vi "Translator.File.Order.vi"(8 "error in":errorcluster, 11 "Translation folder":path=path "D:/PL_0125_Sapphire_Automation_branches/SOFTWARE_v1.1-Translation/settings/Translation-Chinese.ini") -> (0 "error out":errorcluster)   [LabVIEW 2010]
uses:
  tma.lib/nlconfig.llb/nlRead Section (str).vi
  tma.lib/nlconfig.llb/nlWrite Section (str).vi
panel:
  out "section names":string[](array[string])
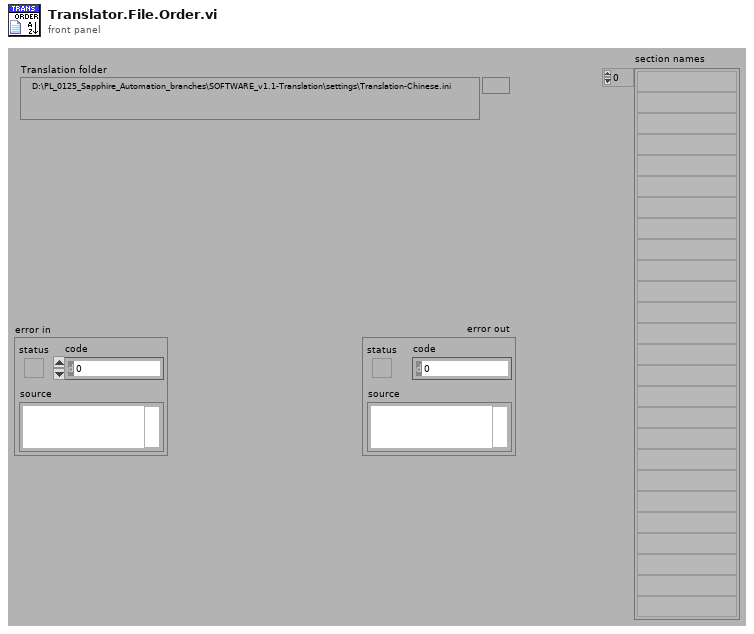
[diagram p1: front panel]
types:
  T1 = typedef "nlConfig Data RefNum.ctl" = refnum<k4>
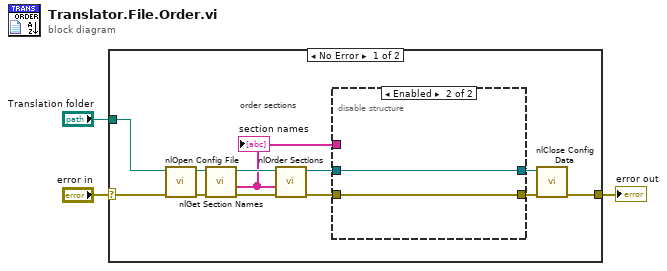
[diagram p0: block diagram]
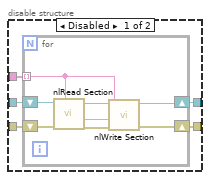
[diagram p2: hidden frame]
diagram:
  n1 = case shown="No Error" "error in" {
    selector: "error in" -> [w10 w31]
    tunnel: "Translation folder" -> [w11 _]
    tunnel: [w9 w31] -> w2
    frame No Error {
      # "order sections"
      n2 = call "nlOpen Config File.vi"("error in (no error)"=w10, "configuration file path"=w11) -> ("error out"=w12:errorcluster, "refnum"=w13:T1)  [unwired: 8 in]
      n3 = call "nlGet Section Names.vi"("error in (no error)"=w12, "refnum"=w13) -> ("error out"=w14:errorcluster, "section names"=w5:string[], "refnum out"=w15:T1)  [unwired: 7 in]
      "section names" <- w5
      n4 = call "nlOrder Sections.vi"("error in (no error)"=w14, "section names"=w5, "refnum"=w15) -> ("error out"=w8:errorcluster, "refnum out"=w7:T1)  [unwired: 7 in]
      n5 = disable-structure shown="Enabled" {
        disable-tunnel: w8 -> [w20 w29]
        disable-tunnel: w7 -> [w19 w30]
        disable-tunnel: [w18 w30] -> w6
        disable-tunnel: w5 -> [w17 _]
        disable-tunnel: [w16 w29] -> w4
        frame Disabled {
          n6 = for {
            tunnel: w17 -> [w23] mode=indexing
            shift-right: [w21] -> w18
            shift-left: w19 -> [w27]
            shift-right: [w22] -> w16
            shift-left: w20 -> [w28]
            n7 = call-poly "nlRead Section.vi"("sectionname"=w23, "error in (no error)"=w28, "refnum"=w27) -> ("error out"=w26:errorcluster, "contents out"=w25:string, "refnum out"=w24:T1)  [unwired: 5 in, 1 out]
            n8 = call-poly "nlWrite Section.vi"("sectionname"=w23, "error in (no error)"=w26, "contents in"=w25, "refnum"=w24) -> ("error out"=w22:errorcluster, "refnum out"=w21:T1)  [unwired: 5 in, 1 out]
          }
        }
        frame Enabled {
        }
      }
      n9 = call "nlClose Config Data.vi"("error in (no error)"=w4, "refnum"=w6) -> ("error out"=w9:errorcluster)  [unwired: 8 in, 1 out]
    }
    frame Error {
    }
  }
  "error out" <- w2
